vi "lsl set value.vi"(8 "error in (no error)":errorcluster, 10 "rhs":string, 11 "e":cluster{}) -> (0 "error out":errorcluster, 2 "function return":i32, 3 "e out":cluster{})   [LabVIEW 2018, in "liblsl-LabVIEW.lvlib"]
doc: "extern LIBLSL_C_API int32_t lsl_set_value(lsl_xml_ptr e, const char *rhs);"
uses:
  <userlib>/liblsl-LabVIEW/liblsl-LabVIEW.lvlib
  <userlib>/liblsl-LabVIEW/liblsl64.dll
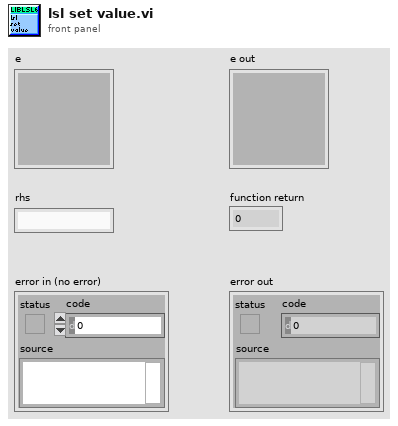
[diagram p1: front panel]
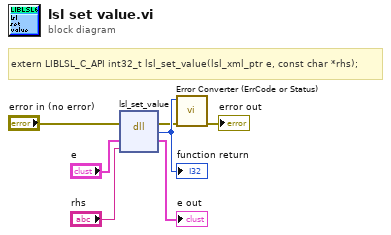
[diagram p0: block diagram]
diagram:
  # "extern LIBLSL_C_API int32_t lsl_set_value(lsl_xml_ptr e, const char *rhs);"
  n1 = dll-call lib="C:/Program Files/National Instruments/LabVIEW 2018/user.lib/liblsl-LabVIEW/liblsl64.*" fn="lsl_set_value"(error in="error in (no error)", "e"="e", "rhs"="rhs") -> (error out=w2:errorcluster, w7:i32, "e"=→"e out":cluster{})  [unwired: 3 in, 1 out]
  "function return" <- w7
  n2 = call <userlib>:"Error Converter (ErrCode or Status).vi"("error in (no error)"=w2, "error code"=w7) -> ("error out"=→"error out":errorcluster)  [unwired: 9 in]
